vi "Main_Host - Initialize Main Paths.vi"(8 "error in (no error)":errorcluster) -> (0 "error out":errorcluster, 3 "Config Files Folder Path":path, 5 "is EXE?":bool)   [LabVIEW 2020]
doc: "JSMA Project Wizard 0.2.0.11\nRob Humfeld - JET Engineering\nCopyright (c) 2020, JET Engineering"
uses:
  <userlib>/JET Engineering/JET File-Dir-Path/File - ReadWrite Permission.vi
  <vilib>/Utility/libraryn.llb/Recursive File List.vi
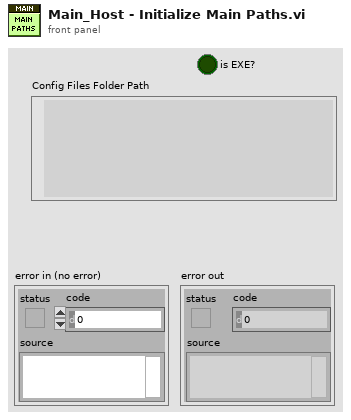
[diagram p1: front panel]
types:
  T1 = enum32{"invalid app kind", "Development System", "Run Time System", "Student Edition", "Embedded LabVIEW", "Evaluation", "Custom"}
  T2 = enum32{"Invalid", "Standard", "Closed", "Hidden", "Minimized", "Maximized"}
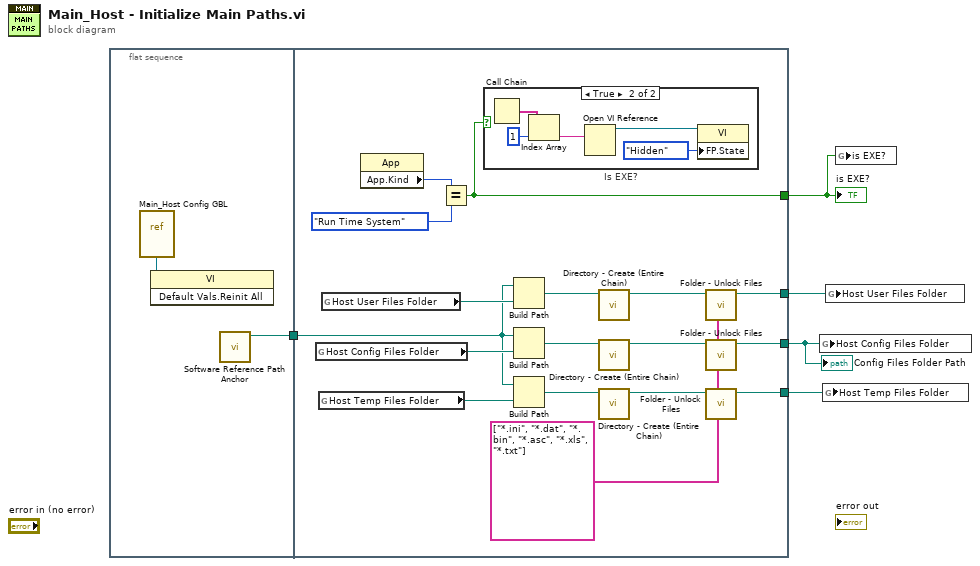
[diagram p0: block diagram]
diagram:
  n1 = flat-sequence {
    tunnel: [w6] -> w2
    tunnel: [w22] -> w5
    tunnel: [w16] -> w4
    tunnel: [w14] -> w3
    tunnel: w2 -> [w10]
    tunnel: [w8] -> w1
    frame #0 {
      n2 = vi-ref "Main_Host Config GBL.vi"() -> (w7:refnum<vi>)
      n3 = invoke class="VI" method="Default Vals.Reinit All"(reference=w7) -> ()  [unwired: 2 in, 3 out]
      n4 = call "Software Reference Path Anchor.vi"() -> ("Reference Directory Path: Software"=w6:path)  [unwired: 11 in]
    }
    frame #1 {
      w9 = string[] ["*.ini", "*.dat", "*.bin", "*.asc", "*.xls", "*.txt"] ("Extensions (*.ini, *.dat, *.bin, *.asc, *.xls)")
      n5 = global read "Main_Host Config GBL.vi" "Host Config Files Folder"() -> (w20:path)
      n6 = global read "Main_Host Config GBL.vi" "Host Temp Files Folder"() -> (w21:path)
      n7 = global read "Main_Host Config GBL.vi" "Host User Files Folder"() -> (w11:path)
      n8 = property class="App"() -> ("App.Kind"=w24:T1)  [unwired: 2 in, 2 out]
      n9 = Equal?(x=w24, y=T1."Run Time System" ("Application:Kind")) -> (x = y?=w22:bool)
      n10 = case "Is EXE?" shown="True" w22 {
        frame False {
        }
        frame True {
          n11 = Call Chain() -> (call chain=w29:string[])
          n12 = Index Array(array=w29, index=1) -> (element=w27:string)
          n13 = Open VI Reference(vi path=w27) -> (vi reference=w26:refnum<vi>)  [unwired: 5 in, 1 out]
          n14 = property class="VI"(reference=w26, "FP.State"=T2."Hidden" ("Front Panel Window:State")) -> ()  [unwired: 1 in, 2 out]
        }
      }
      n15 = Build Path(base path=w10, name or relative path=w11) -> (appended path=w12:path)
      n16 = Build Path(base path=w10, name or relative path=w20) -> (appended path=w18:path)
      n17 = Build Path(base path=w10, name or relative path=w21) -> (appended path=w19:path)
      n18 = call <userlib>:"Directory - Create (Entire Chain).vi"("Directory path"=w12) -> ("Directory path [copy]"=w13:path)  [unwired: 9 in, 1 out]
      n19 = call <userlib>:"Directory - Create (Entire Chain).vi"("Directory path"=w18) -> ("Directory path [copy]"=w17:path)  [unwired: 9 in, 1 out]
      n20 = call <userlib>:"Directory - Create (Entire Chain).vi"("Directory path"=w19) -> ("Directory path [copy]"=w15:path)  [unwired: 9 in, 1 out]
      n21 = call <userlib>:"Folder - Unlock Files.vi"("Extensions (*.ini, *.dat, *.bin, *.asc, *.xls)"=w9, "Directory path"=w13) -> ("Directory path"=w8:path)  [unwired: 9 in]
      n22 = call <userlib>:"Folder - Unlock Files.vi"("Extensions (*.ini, *.dat, *.bin, *.asc, *.xls)"=w9, "Directory path"=w17) -> ("Directory path"=w16:path)  [unwired: 9 in]
      n23 = call <userlib>:"Folder - Unlock Files.vi"("Extensions (*.ini, *.dat, *.bin, *.asc, *.xls)"=w9, "Directory path"=w15) -> ("Directory path"=w14:path)  [unwired: 9 in]
    }
  }
  n24 = global write "Main_Host Config GBL.vi" "Host Config Files Folder"(w4) -> ()
  n25 = global write "Main_Host Config GBL.vi" "Host Temp Files Folder"(w3) -> ()
  n26 = global write "Main_Host Config GBL.vi" "Host User Files Folder"(w1) -> ()
  n27 = global write "Main_Host Config GBL.vi" "is EXE?"(w5) -> ()
  "Config Files Folder Path" <- w4
  "is EXE?" <- w5
